vi "determineSubDataSVs.vi"(8 "error in (no error)":errorcluster, 11 "DataListenerThisComponent in":refnum<class "DataListenerThisComponent.lvclass">) -> (0 "error out":errorcluster, 2 "svNames":string[](array[string]), 3 "DataListenerThisComponent out":refnum<class "DataListenerThisComponent.lvclass">)   [LabVIEW 2012, in "DataListenerThisComponent.lvclass"]
uses:
  DataListenerThisComponent.lvclass
  Typedefs/SubDataSV.ctl
  DataListenerThisComponent.lvclass/DataListenerThisComponent.ctl
  Typedefs/EXATypedefs.lvlib
  <vilib>/Utility/VariantDataType/VariantType.lvlib
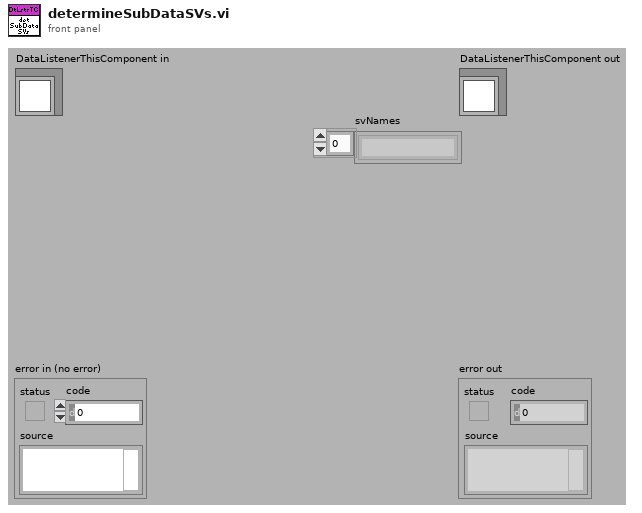
[diagram p1: front panel]
types:
  T1 = typedef "EXATypedefs.lvlib/SubDataSV.ctl" = enum16{"ClearError", "Disable", "Enable", "Exit", "GoToStandby", "HeartbeatIn", "Start"}
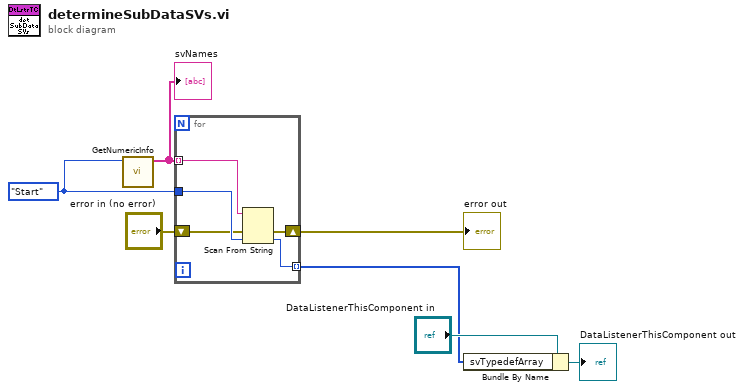
[diagram p0: block diagram]
diagram:
  w7 = SubDataSV."Start" ("SubDataSV")
  n1 = call <vilib>:"GetNumericInfo.vi"("Variant"=w7) -> ("EnumNames"=w3:string[])  [unwired: 7 in, 3 out]
  "svNames" <- w3
  n2 = for {
    tunnel: [w11] -> w4 mode=indexing
    shift-right: [w9] -> w1
    shift-left: "error in (no error)" -> [w10]
    tunnel: w3 -> [w8] mode=indexing
    tunnel: w7 -> [w12]
    n3 = Scan From String(input string=w8, error in=w10, default 1=w12) -> (error out=w9:errorcluster, output 1=w11:T1)  [unwired: 2 in, 2 out]
  }
  "error out" <- w1
  n4 = Bundle By Name(cluster="DataListenerThisComponent in", "svTypedefArray"=w4) -> (→"DataListenerThisComponent out":refnum<class "DataListenerThisComponent.lvclass">)
